vi "Engine - Close HW.vi"(8 "error in (no error)":errorcluster, 10 "DMM Ref In":refnum<k15>, 11 "SWITCH Ref In":refnum<k15>) -> (0 "error out":errorcluster)   [LabVIEW 2016, in "DMM-SWITCH-ScanList Engine.lvlib"]
doc: "Abort tasks and close references for Switch and DMM devices"
uses:
  DMM-SWITCH-ScanList Engine.lvlib
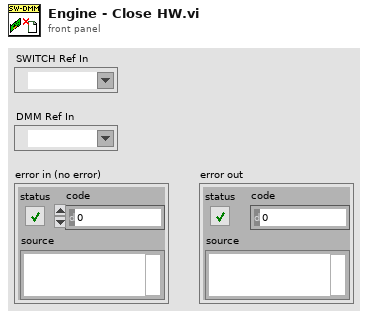
[diagram p1: front panel]
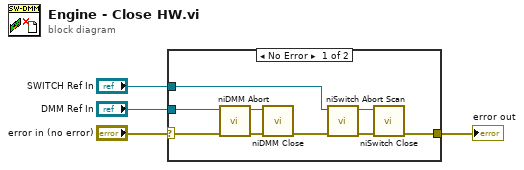
[diagram p0: block diagram]
diagram:
  n1 = case shown="No Error" "error in (no error)" {
    selector: "error in (no error)" -> [w5 w14]
    tunnel: "SWITCH Ref In" -> [w13 _]
    tunnel: "DMM Ref In" -> [w12 _]
    tunnel: [w11 w14] -> w2
    frame No Error {
      n2 = call <instrlib>:"niDMM Abort.vi"("error in (no error)"=w5, "instrument handle"=w12) -> ("error out"=w7:errorcluster, "instrument handle out"=w8:refnum<k15>)  [unwired: 8 out]
      n3 = call <instrlib>:"niDMM Close.vi"("error in (no error)"=w7, "instrument handle"=w8) -> ("error out"=w6:errorcluster)  [unwired: 9 out]
      n4 = call <instrlib>:"niSwitch Abort Scan.vi"("error in (no error)"=w6, "instrument handle"=w13) -> ("error out"=w9:errorcluster, "instrument handle out"=w10:refnum<k15>)  [unwired: 8 out]
      n5 = call <instrlib>:"niSwitch Close.vi"("error in (no error)"=w9, "instrument handle"=w10) -> ("error out"=w11:errorcluster)  [unwired: 9 out]
    }
    frame Error {
    }
  }
  "error out" <- w2
